vi "X-_mnemonics.vi"(0 "COMMAND":T1) -> (1 "Mnemonic":string, 2 "Readable":bool, 3 "Writeable":bool)   [LabVIEW 2010]
uses:
  X-_commands.ctl
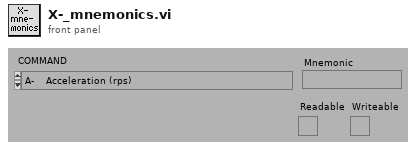
[diagram p1: front panel]
types:
  T1 = typedef "X-_commands.ctl" = enum16{"A-    Acceleration (rps)", "B-    Buffer Status", "C-    Continue", "CG-  Correction Gain", "CR-  Cariage Return", "D-    Distance (pulses)", "DB-  Dead Band (encoder steps)", "DW- Deadband Window (encoder steps)", "E-    Enable Communications", "ER-  Encoder Resolution (steps/rev)", "F-    Disable Communications", "FS-  Encoder Functions Report", "FSA- Incremental/Absolute (0/1)", "FSB- Motor/Encoder Step Mode (0/1)", "FSC- Enable/Disable Position Maint. (1/0)", "FSD- Stop/Continue on Stall (1/0)", "FSE- Activate o/p1 on Stall (1/0)", "FSF- Stop Motion on Trig3 (1/0)", "FSG- Activate o/p2 in Deadband (1/0)", "FSH- Enable Stall Detect (1/0)", "G- Go", "GH- Go Home and Zero (+/-V)", "^H- Delete ", "H- Direction Reverse/CCW/CW (0,1,2)", "IS- Input Status", "K- Kill", "L- Loop (n)", "LD- Limit DISABLE (0-none,1-CW,2-CCW,3-Both)", "LF- Line Feed", "MC- Mode Continuous", "MN- Mode Normal", "MPA- Motor Postion Absolute", "MPI- Motor Position Incremental", "MR- Motor Resolution (Drive Steps/rev)", "N- End of Loop", "O- Output (00,01,10,11)", "OS- Report Homing Setup", "OSA- NO/NC Limits (1/0)", "OSB- Back Up to Home/Edge? (0/1)", "OSC- NO/NC Home Switch (1/0)", "OSD- Enable Encoder Z for Home (0/1)", "OSH- Reference Edge for Home CW/CCW (0/1)", "PR- Report ABSOLUTE Position", "PS- Pause until Continue", "PX- Report Absolute ENCODER Position", "PZ- Zero Absolute Counter", "\"- Quote (17 ASCII +Space)", "Q- Enter/Exit Velocity Profiling (1/0)", "R- Request Indexer Status", "RA- Report Limit Switch Status", "RB- Report Loop, Pause, Shutdown, Trigger Status", "RC- Report Closed Loop Status", "RM- Velocity Streaming Rate Multiplier (000-FFF)", "RV- Report Revision Level", "S- Controlled Stop", "SN- Debounce (1-1000ms)", "SS- Report Software Switch Status", "SSA- Disable RS232 Echo (1/0)", "SSG- Clear/Save Command Buffer on Limit (0/1)", "SSH- Clear/Save Command Buffer on Stop (0/1)", "ST- Shutdown (1/0)", "SV- Servoing Setting (0,1,2,3)", "T- Time Delay (0.01-99999.99)", "TR- Wait for Trigger High/Low/Ignore (1/0/X)", "TS- Report Trigger Status", "U- Pause after Move Until Continue", "V- Velocity (0.01-50.00 revs/sec)", "W1- Report Relative Position <Signed Binary>", "W3- Report Relative Position <Hexadecimal>", "Y- Abort Loop at N", "Z-    Reset to Defaults", "#-    Disable/Set Soft Addresses (0/1-255)"}
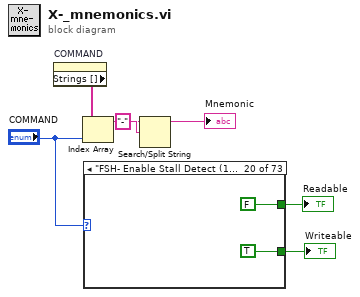
[diagram p0: block diagram]
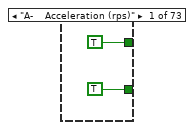
[diagram p2: hidden frame]
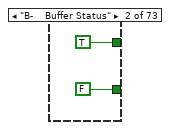
[diagram p3: hidden frame]
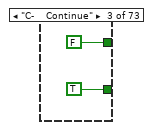
[diagram p4: hidden frame]
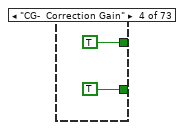
[diagram p5: hidden frame]
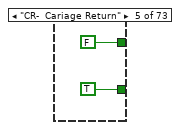
[diagram p6: hidden frame]
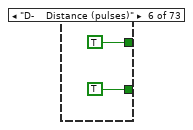
[diagram p7: hidden frame]
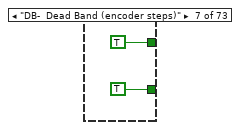
[diagram p8: hidden frame]
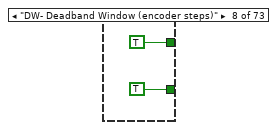
[diagram p9: hidden frame]
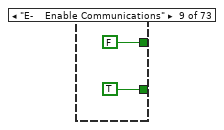
[diagram p10: hidden frame]
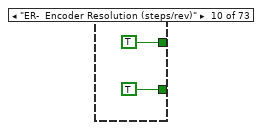
[diagram p11: hidden frame]
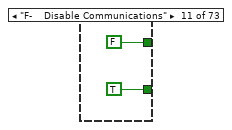
[diagram p12: hidden frame]
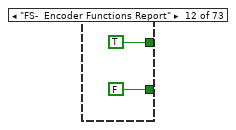
[diagram p13: hidden frame]
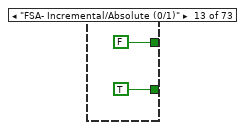
[diagram p14: hidden frame]
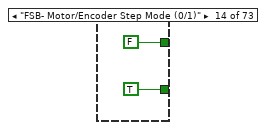
[diagram p15: hidden frame]
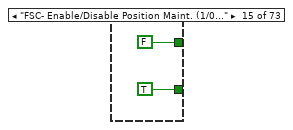
[diagram p16: hidden frame]
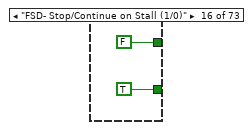
[diagram p17: hidden frame]
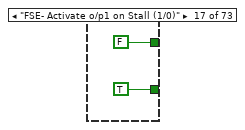
[diagram p18: hidden frame]
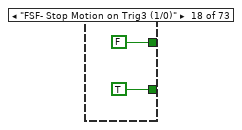
[diagram p19: hidden frame]
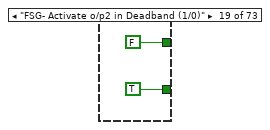
[diagram p20: hidden frame]
diagram:
  n1 = property on="COMMAND" class="Enum (strict)"() -> ("Strings []"=w4:string[])  [unwired: 2 in, 2 out]
  n2 = Index Array(array=w4, index="COMMAND") -> (element=w5:string)
  n3 = case shown="\"FSH- Enable Stall Detect (1/0)\"" "COMMAND" {
    tunnel: [TRUE TRUE FALSE TRUE FALSE TRUE TRUE TRUE FALSE TRUE FALSE TRUE FALSE FALSE FALSE FALSE FALSE FALSE FALSE FALSE FALSE FALSE FALSE FALSE TRUE FALSE FALSE FALSE FALSE FALSE FALSE FALSE FALSE TRUE FALSE FALSE TRUE FALSE FALSE FALSE FALSE FALSE TRUE FALSE TRUE FALSE FALSE FALSE TRUE TRUE TRUE TRUE FALSE TRUE FALSE TRUE TRUE FALSE FALSE FALSE FALSE TRUE FALSE FALSE TRUE FALSE TRUE TRUE TRUE FALSE FALSE FALSE FALSE] -> w3
    tunnel: [TRUE FALSE TRUE TRUE TRUE TRUE TRUE TRUE TRUE TRUE TRUE FALSE TRUE TRUE TRUE TRUE TRUE TRUE TRUE TRUE TRUE TRUE TRUE TRUE FALSE TRUE TRUE TRUE TRUE TRUE TRUE TRUE TRUE TRUE TRUE TRUE FALSE TRUE TRUE TRUE TRUE TRUE FALSE TRUE FALSE TRUE TRUE TRUE FALSE FALSE FALSE FALSE TRUE FALSE TRUE TRUE FALSE TRUE TRUE TRUE TRUE TRUE TRUE TRUE FALSE TRUE TRUE FALSE FALSE TRUE TRUE TRUE FALSE] -> w2
    frame "A-    Acceleration (rps)" {
    }
    frame "B-    Buffer Status" {
    }
    frame "C-    Continue" {
    }
    frame "CG-  Correction Gain" {
    }
    frame "CR-  Cariage Return" {
    }
    frame "D-    Distance (pulses)" {
    }
    frame "DB-  Dead Band (encoder steps)" {
    }
    frame "DW- Deadband Window (encoder steps)" {
    }
    frame "E-    Enable Communications" {
    }
    frame "ER-  Encoder Resolution (steps/rev)" {
    }
    frame "F-    Disable Communications" {
    }
    frame "FS-  Encoder Functions Report" {
    }
    frame "FSA- Incremental/Absolute (0/1)" {
    }
    frame "FSB- Motor/Encoder Step Mode (0/1)" {
    }
    frame "FSC- Enable/Disable Position Maint. (1/0)" {
    }
    frame "FSD- Stop/Continue on Stall (1/0)" {
    }
    frame "FSE- Activate o/p1 on Stall (1/0)" {
    }
    frame "FSF- Stop Motion on Trig3 (1/0)" {
    }
    frame "FSG- Activate o/p2 in Deadband (1/0)" {
    }
    frame "FSH- Enable Stall Detect (1/0)" {
    }
    frame "G- Go" {
    }
    frame "GH- Go Home and Zero (+/-V)" {
    }
    frame "^H- Delete " {
    }
    frame "H- Direction Reverse/CCW/CW (0,1,2)" {
    }
    frame "IS- Input Status" {
    }
    frame "K- Kill" {
    }
    frame "L- Loop (n)" {
    }
    frame "LD- Limit DISABLE (0-none,1-CW,2-CCW,3-Both)" {
    }
    frame "LF- Line Feed" {
    }
    frame "MC- Mode Continuous" {
    }
    frame "MN- Mode Normal" {
    }
    frame "MPA- Motor Postion Absolute" {
    }
    frame "MPI- Motor Position Incremental" {
    }
    frame "MR- Motor Resolution (Drive Steps/rev)" {
    }
    frame "N- End of Loop" {
    }
    frame "O- Output (00,01,10,11)" {
    }
    frame "OS- Report Homing Setup" {
    }
    frame "OSA- NO/NC Limits (1/0)" {
    }
    frame "OSB- Back Up to Home/Edge? (0/1)" {
    }
    frame "OSC- NO/NC Home Switch (1/0)" {
    }
    frame "OSD- Enable Encoder Z for Home (0/1)" {
    }
    frame "OSH- Reference Edge for Home CW/CCW (0/1)" {
    }
    frame "PR- Report ABSOLUTE Position" {
    }
    frame "PS- Pause until Continue" {
    }
    frame "PX- Report Absolute ENCODER Position" {
    }
    frame "PZ- Zero Absolute Counter" {
    }
    frame "\"- Quote (17 ASCII +Space)" {
    }
    frame "Q- Enter/Exit Velocity Profiling (1/0)" {
    }
    frame "R- Request Indexer Status" {
    }
    frame "RA- Report Limit Switch Status" {
    }
    frame "RB- Report Loop, Pause, Shutdown, Trigger Status" {
    }
    frame "RC- Report Closed Loop Status" {
    }
    frame "RM- Velocity Streaming Rate Multiplier (000-FFF)" {
    }
    frame "RV- Report Revision Level" {
    }
    frame "S- Controlled Stop" {
    }
    frame "SN- Debounce (1-1000ms)" {
    }
    frame "SS- Report Software Switch Status" {
    }
    frame "SSA- Disable RS232 Echo (1/0)" {
    }
    frame "SSG- Clear/Save Command Buffer on Limit (0/1)" {
    }
    frame "SSH- Clear/Save Command Buffer on Stop (0/1)" {
    }
    frame "ST- Shutdown (1/0)" {
    }
    frame "SV- Servoing Setting (0,1,2,3)" {
    }
    frame "T- Time Delay (0.01-99999.99)" {
    }
    frame "TR- Wait for Trigger High/Low/Ignore (1/0/X)" {
    }
    frame "TS- Report Trigger Status" {
    }
    frame "U- Pause after Move Until Continue" {
    }
    frame "V- Velocity (0.01-50.00 revs/sec)" {
    }
    frame "W1- Report Relative Position <Signed Binary>" {
    }
    frame "W3- Report Relative Position <Hexadecimal>" {
    }
    frame "Y- Abort Loop at N" {
    }
    frame "Z-    Reset to Defaults" {
    }
    frame "#-    Disable/Set Soft Addresses (0/1-255)" {
    }
    frame Default {
    }
  }
  "Readable" <- w3
  "Writeable" <- w2
  n4 = Search/Split String(string=w5, search string/char (-)="-" ("search char (-)")) -> (substring before match=→"Mnemonic":string)  [unwired: 3 out]
